vi "test_rozptyl.vi"() -> ()   [LabVIEW 2024]
uses:
  <vilib>/Analysis/baseanly.llb/Mean (DBL).vi
  <instrlib>/EFmeter/Public/Data/Read (Single Point).vi
  <instrlib>/EFmeter/EFmeter.lvlib
  <vilib>/Analysis/NI_AALBase.lvlib
panel:
  in  "Cancel Button":bool
  out "Waveform Chart":dbl[](graph)
  in  "VISA EFmeter":refnum<visa-resource-name>
  in  "file path (use dialog)":path
  in  "Prumerovani":bool
  in  "Vzorku na krokù":u16 max=100 step=1
  in  "Combo Box":string(combo)="VOLT"
  in  "Ring":u16(ring)=1 items=["CH2"=2, "CH1"=1]
  in  "Clear":bool
  in  "Uložit data":bool
  in  "vyh\nVyhodnotit":bool
  in  "Další":bool caption="OK Button"
  in  "Start":bool
  in  "stop":bool
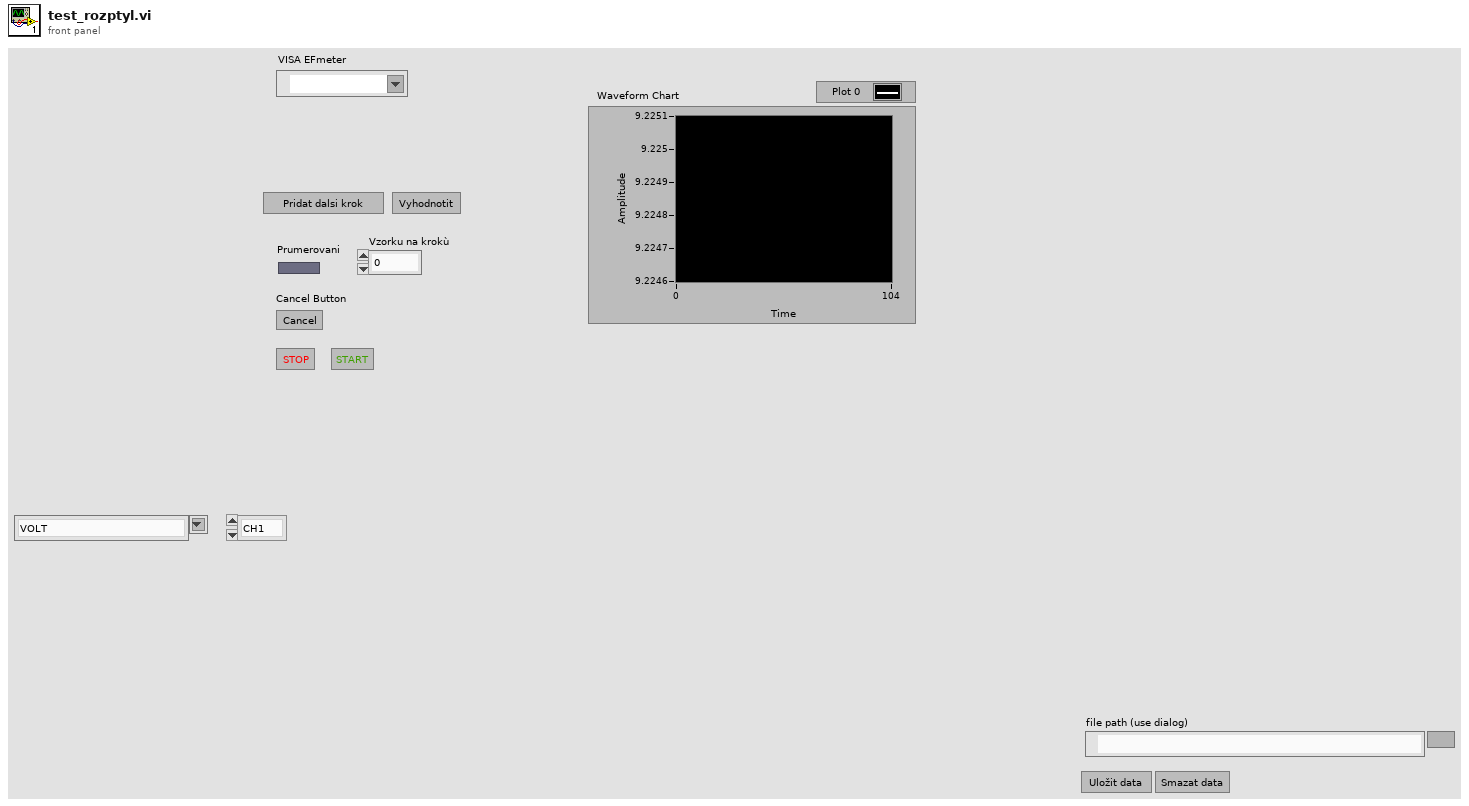
[diagram p1: front panel]
types:
  T1 = enum16{"init", "wait", "graph", "meas", "change_load", "init_measurment", "save", "clear"}
  T2 = enum16{"open", "replace", "create", "open or create", "replace or create", "replace or create with confirmation"}
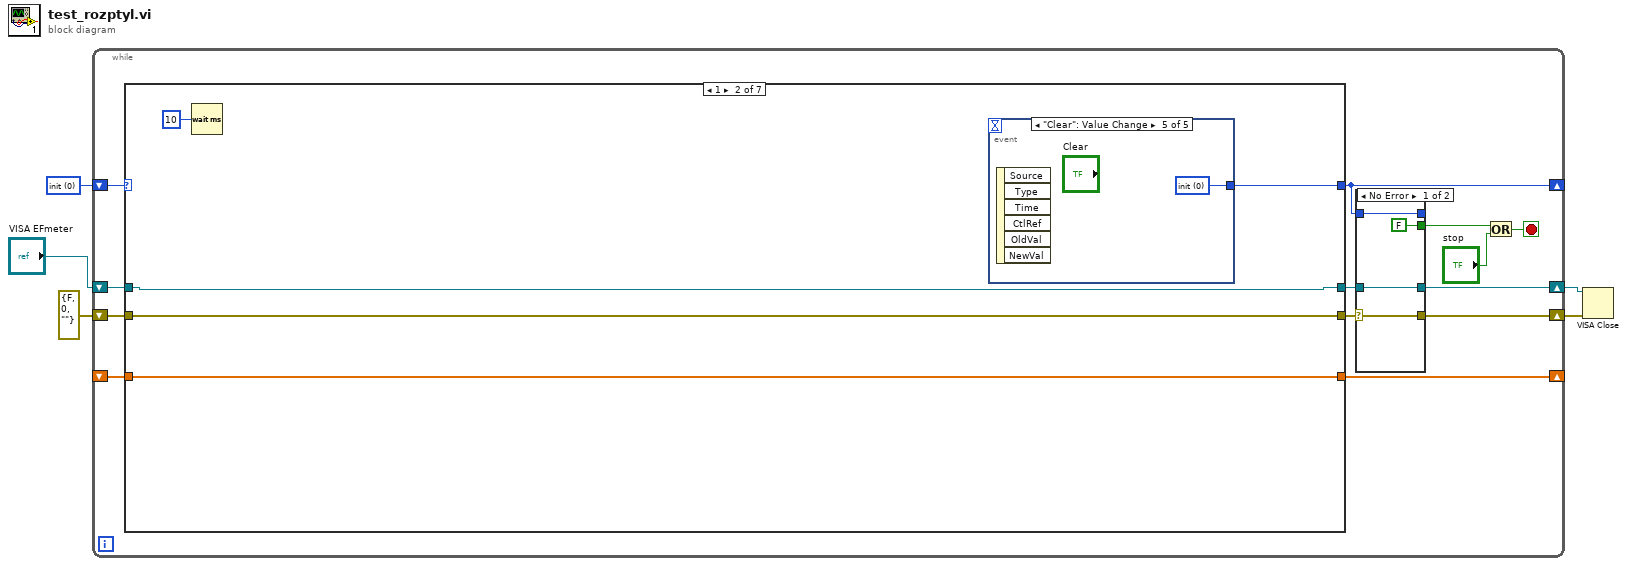
[diagram p0: block diagram]
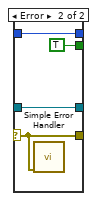
[diagram p2: hidden frame]
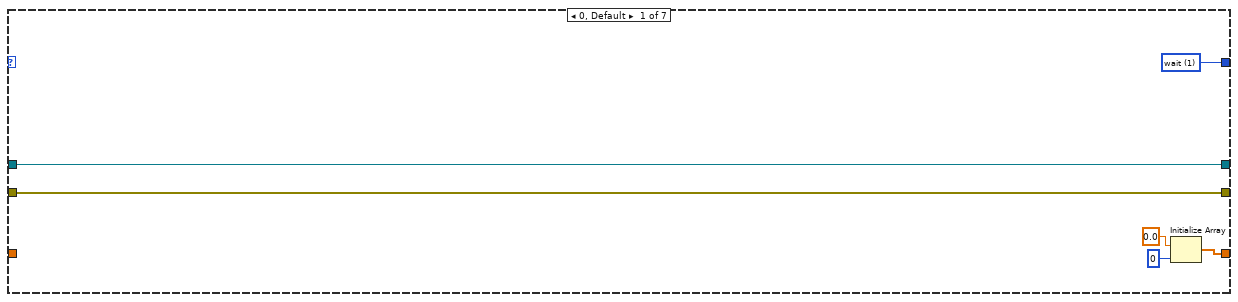
[diagram p3: hidden frame]
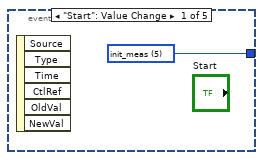
[diagram p4: hidden frame]
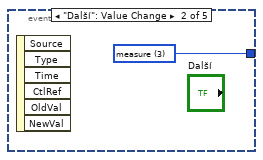
[diagram p5: hidden frame]
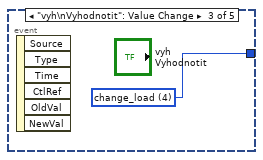
[diagram p6: hidden frame]
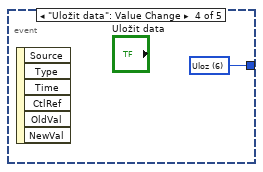
[diagram p7: hidden frame]
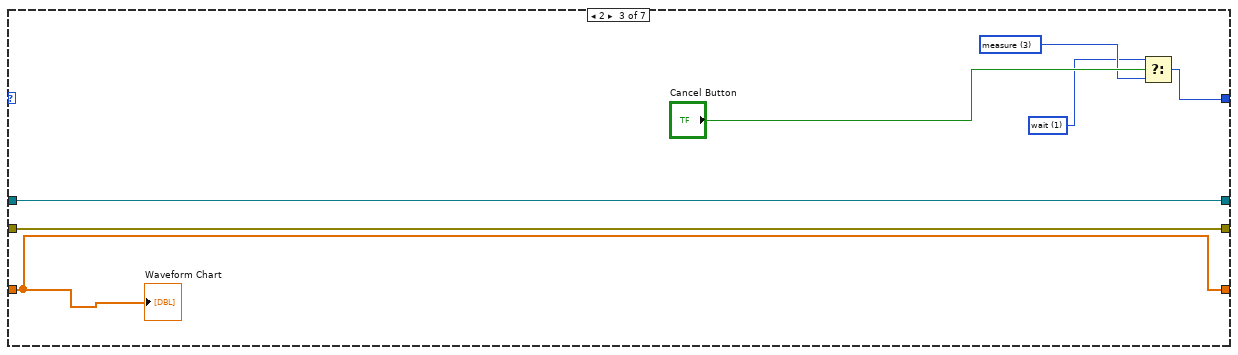
[diagram p8: hidden frame]
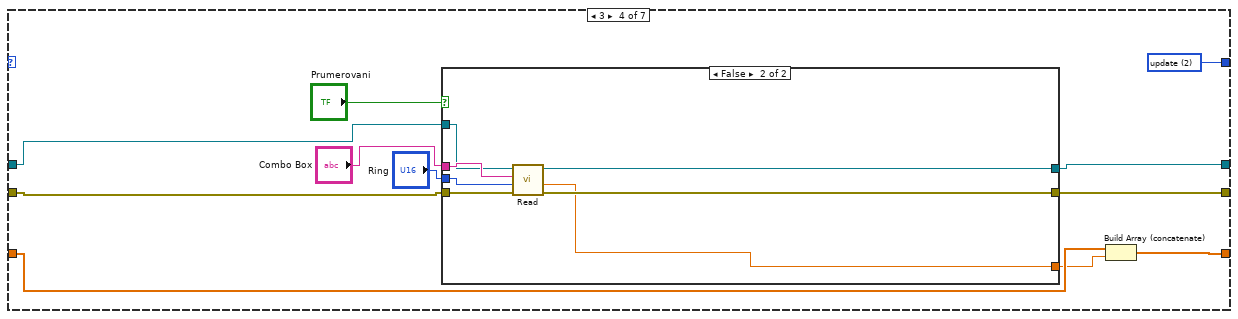
[diagram p9: hidden frame]
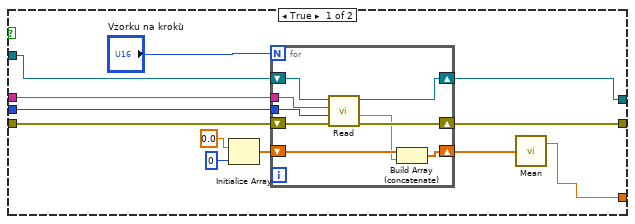
[diagram p10: hidden frame]
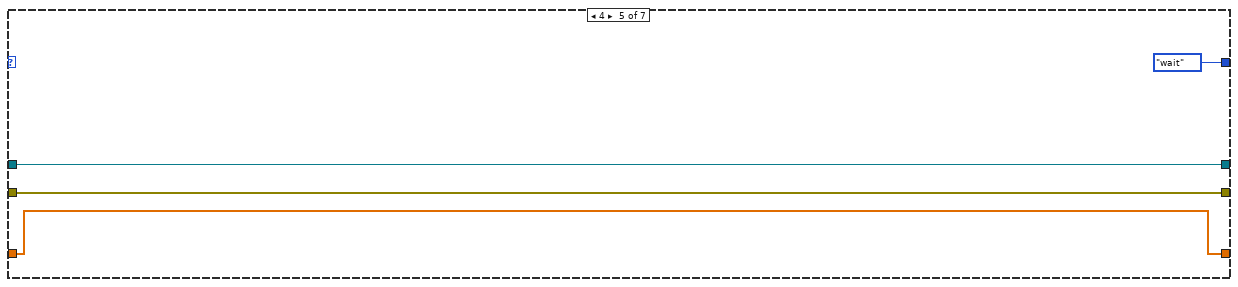
[diagram p11: hidden frame]
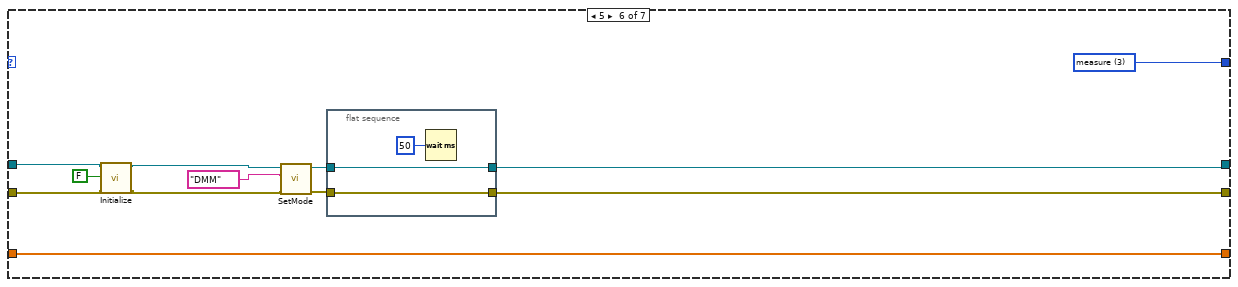
[diagram p12: hidden frame]
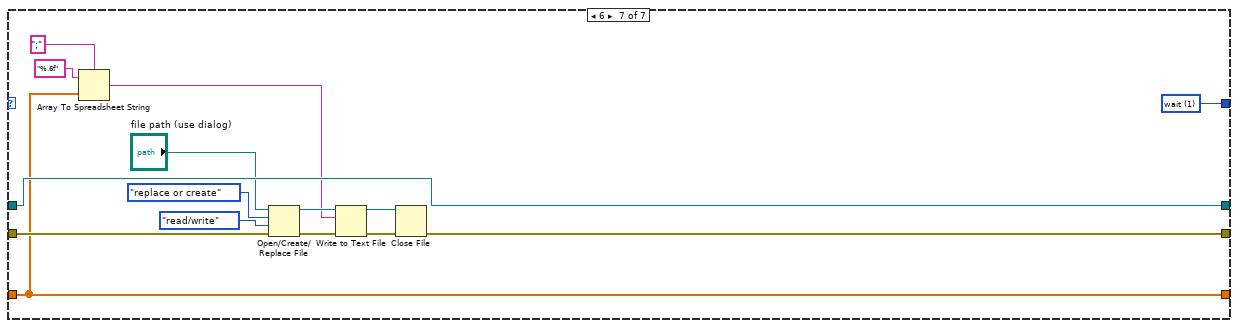
[diagram p13: hidden frame]
diagram:
  w5 = u16 0 items=["init", "wait", "update", "measure", "change_load", "init_meas", "Uloz", "clear"]
  n1 = while {
    shift-right: [w18] -> _
    shift-left: _ -> [w6]
    shift-right: [w14] -> _
    shift-left: w5 -> [w17]
    shift-right: [w11] -> w2
    shift-left: "VISA EFmeter" -> [w16]
    shift-right: [w10] -> w1
    shift-left: errorcluster {"status"=FALSE, "code"=0, "source"=""} ("error in (no error)") -> [w15]
    stop <- w8 stop-if-true
    n2 = case shown="1" w17 {
      tunnel: [w30 w33 w47 w60 w89 w101 w108] -> w18
      tunnel: [w29 w37 w43 w59 T1."wait" w104 w116] -> w14
      tunnel: [w27 w35 w48 w55 w90 w102 w112] -> w13
      tunnel: [w28 w36 w49 w56 w92 w103 w122] -> w12
      tunnel: w16 -> [w28 w36 w49 w58 w92 w99 w122]
      tunnel: w15 -> [w27 w35 w48 w57 w90 w98 w118]
      tunnel: w6 -> [_ w33 w47 w53 w89 w101 w108]
      frame 0, Default {
        w29 = u16 1 items=["init", "wait", "update", "measure"]
        n3 = Initialize Array(0.0 ("element"), 0 ("dimension size")) -> (w30:dbl[])
      }
      frame 1 {
        n4 = Wait (ms)(milliseconds to wait=u32 10) -> ()  [unwired: 1 out]
        n5 = event shown="[4] \"Clear\": Value Change" {
          selector: _ -> [_ _ _ _ _]
          dyn-events: _ -> [_ _ _ _ _]
          timeout: _ -> [_ _ _ _ _]
          tunnel: [w38 w39 w40 w41 w42] -> w37
          event "Start": Value Change {
            w38 = u16 5 items=["init", "wait", "update", "measure", "change_load", "init_meas"]
            n6 = event-data() -> ()  [unwired: 1 in, 6 out]
          }
          event "Další": Value Change {
            w39 = u16 3 items=["init", "wait", "update", "measure", "change_load", "init_meas", "Uloz", "clear"]
            n7 = event-data() -> ()  [unwired: 1 in, 6 out]
          }
          event "vyh\nVyhodnotit": Value Change {
            w40 = u16 4 items=["init", "wait", "update", "measure", "change_load", "init_meas", "Uloz", "clear"]
            n8 = event-data() -> ()  [unwired: 1 in, 6 out]
          }
          event "Uložit data": Value Change {
            w41 = u16 6 items=["init", "wait", "update", "measure", "change_load", "init_meas", "Uloz"]
            n9 = event-data() -> ()  [unwired: 1 in, 6 out]
          }
          event "Clear": Value Change {
            w42 = u16 0 items=["init", "wait", "update", "measure", "change_load", "init_meas", "Uloz", "clear"]
            n10 = event-data() -> ()  [unwired: 1 in, 6 out]
          }
        }
      }
      frame 2 {
        w44 = u16 1 items=["init", "wait", "update", "measure"]
        w45 = u16 3 items=["init", "wait", "update", "measure"]
        n11 = Select(t=w44, s="Cancel Button", f=w45) -> (s? t:f=w43:u16)
        "Waveform Chart" <- w47
      }
      frame 3 {
        w59 = u16 2 items=["init", "wait", "update", "measure"]
        n12 = case shown="False" "Prumerovani" {
          tunnel: w58 -> [w68 w85]
          tunnel: w57 -> [w67 w88]
          tunnel: [w66 w84] -> w56
          tunnel: [w65 w83] -> w55
          tunnel: "Combo Box" -> [w63 w86]
          tunnel: "Ring" -> [w62 w87]
          tunnel: [w61 w82] -> w50
          frame True {
            n13 = Initialize Array(0.0 ("element"), 0 ("dimension size")) -> (w69:dbl[])
            n14 = for {
              N: "Vzorku na krokù" -> [_]
              shift-right: [w73] -> w66
              shift-left: w68 -> [w76]
              shift-right: [w75] -> w65
              shift-left: w67 -> [w79]
              shift-right: [w80] -> w64
              shift-left: w69 -> [w81]
              tunnel: w63 -> [w78]
              tunnel: w62 -> [w77]
              n15 = call-poly <instrlib>:"Read.vi"("error in (no error)"=w79, "Ring"=w77, "Combo Box"=w78, "VISA resource name"=w76) -> ("error out"=w75:errorcluster, "Measurement"=w74:dbl, "VISA resource name out"=w73:refnum<visa-resource-name>)  [unwired: 5 in]
              n16 = Build Array (concatenate)(w81, w74) -> (w80:dbl[])
            }
            n17 = call-poly <vilib>:"Mean.vi"("X"=w64) -> ("mean"=w61:dbl)  [unwired: 1 out]
          }
          frame False {
            n18 = call-poly <instrlib>:"Read.vi"("error in (no error)"=w88, "Ring"=w87, "Combo Box"=w86, "VISA resource name"=w85) -> ("error out"=w83:errorcluster, "Measurement"=w82:dbl, "VISA resource name out"=w84:refnum<visa-resource-name>)  [unwired: 5 in]
          }
        }
        n19 = Build Array (concatenate)(w53, w50) -> (w60:dbl[])
      }
      frame 4 {
      }
      frame 5 {
        w104 = u16 3 items=["init", "wait", "update", "measure", "change_load", "init_meas"]
        n20 = call <instrlib>:"Initialize.vi"("error in (no error)"=w98, "ID Query (True)"=FALSE, "VISA resource name"=w99) -> ("error out"=w95:errorcluster, "VISA resource name out"=w93:refnum<visa-resource-name>)  [unwired: 7 in]
        n21 = call <instrlib>:"SetMode.vi"("error in (no error)"=w95, "Combo Box"="DMM", "VISA resource name"=w93) -> ("error out"=w96:errorcluster, "VISA resource name out"=w97:refnum<visa-resource-name>)  [unwired: 7 in]
        n22 = flat-sequence {
          tunnel: [w106] -> w103
          tunnel: w97 -> [w106]
          tunnel: w96 -> [w105]
          tunnel: [w105] -> w102
          frame #0 {
            n23 = Wait (ms)(milliseconds to wait=u32 50) -> ()  [unwired: 1 out]
          }
        }
      }
      frame 6 {
        w116 = u16 1 items=["init", "wait", "update", "measure", "change_load", "init_meas"]
        n24 = Array To Spreadsheet String(delimiter (Tab)=";", array=w108, 3:"%.6f" ("format string")) -> (spreadsheet string=w109:string)
        n25 = Open/Create/Replace File(file path (use dialog)="file path (use dialog)", error in=w118, operation (0:open)=T2."replace or create", access (0:read/write)=enum16{"read/write", "read-only", "write-only"}."read/write") -> (refnum out=w111:refnum<file>, error out=w114:errorcluster)  [unwired: 2 in, 1 out]
        n26 = Write to Text File(file (use dialog)=w111, text=w109, error in=w114) -> (refnum out=w110:refnum<file>, error out=w113:errorcluster)  [unwired: 1 in, 1 out]
        n27 = Close File(refnum=w110, error in=w113) -> (error out=w112:errorcluster)  [unwired: 1 out]
      }
    }
    n28 = case shown="No Error" w13 {
      selector: w13 -> [w20 w23]
      tunnel: w14 -> [w22 w25]
      tunnel: [w22 w25] -> _
      tunnel: w12 -> [w21 w26]
      tunnel: [w21 w26] -> w11
      tunnel: [w20 w23] -> w10
      tunnel: [FALSE TRUE] -> w7
      frame No Error {
      }
      frame Error {
        n29 = call <vilib>:"Simple Error Handler.vi"("error in (no error)"=w23) -> ()  [unwired: 4 in, 5 out]
      }
    }
    n30 = Or(x=w7, y="stop") -> (x .or. y?=w8:bool)
  }
  n31 = VISA Close(VISA resource name=w2, error in (no error)=w1) -> ()  [unwired: 1 out]
